vi "Modify Stage Limits.vi"(0 "Notifier Name":string, 5 "Limits":dbl[][](array[numeric]), 7 "Use Limits?":bool, 11 "Error In":errorcluster) -> (15 "Error Out":errorcluster)   [LabVIEW 2020]
uses:
  Stages Limits Type Defs/Stage Limits.ctl
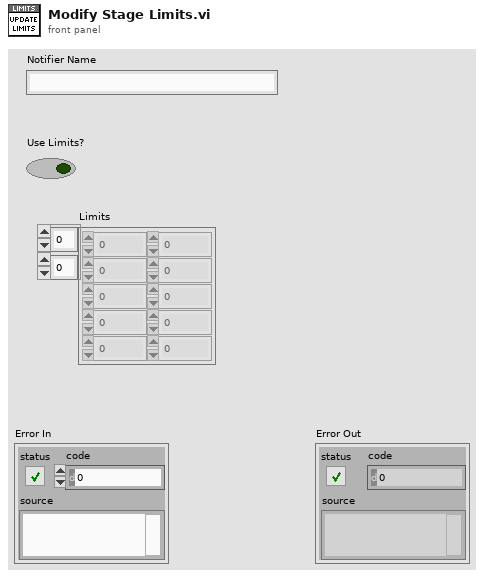
[diagram p1: front panel]
types:
  T1 = typedef "Stage Limits.ctl" = cluster{"Notifier":string, "Use Limits":bool, "Limits":dbl[][]}
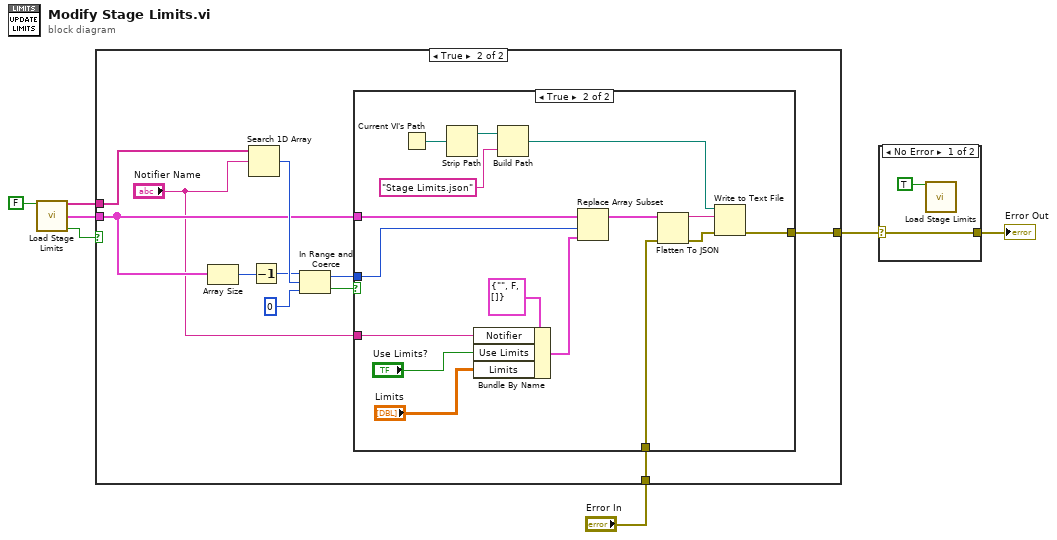
[diagram p0: block diagram]
diagram:
  n1 = call "Load Stage Limits.vi"("Update Limits"=FALSE) -> ("Notifier Names"=w6:string[], "Stage Limits"=w5:T1[], "Loaded"=w4:bool)  [unwired: 12 in]
  n2 = case shown="True" w4 {
    tunnel: w6 -> [_ w19]
    tunnel: w5 -> [_ w12]
    tunnel: [w8 w10] -> w3
    tunnel: "Error In" -> [w8 w9]
    frame False {
    }
    frame True {
      n3 = Array Size(array=w12) -> (size(s)=w16:i32)
      n4 = Search 1D Array(1D array=w19, element="Notifier Name") -> (index of element=w17:i32)  [unwired: 1 in]
      n5 = Decrement(x=w16) -> (x-1=w15:i32)
      n6 = In Range and Coerce(upper limit=w15, x=w17, lower limit=0) -> (coerced(x)=w13:i32, In Range?=w14:bool)
      n7 = case shown="True" w14 {
        tunnel: w13 -> [_ w35]
        tunnel: w12 -> [_ w36]
        tunnel: "Notifier Name" -> [_ w32]
        tunnel: [w20 w22] -> w10
        tunnel: w9 -> [w20 w21]
        frame False {
        }
        frame True {
          n8 = Current VI's Path() -> (path=w26:path)
          n9 = Strip Path(path=w26) -> (stripped path=w25:path)  [unwired: 1 out]
          n10 = Bundle By Name(cluster=T1 {"Notifier"="", "Use Limits"=FALSE, "Limits"=[]} ("Stage Limits"), "Notifier"=w32, "Use Limits"="Use Limits?", "Limits"="Limits") -> (w33:T1)
          n11 = Build Path(base path=w25, name or relative path="Stage Limits.json") -> (appended path=w23:path)
          n12 = Replace Array Subset(array=w36, new element=w33, index=w35) -> (w28:T1[])
          n13 = Flatten To JSON(anything=w28, error in (no error)=w21) -> (JSON string=w29:string, 11:w27:errorcluster)  [unwired: 1 in]
          n14 = Write to Text File(file (use dialog)=w23, text=w29, error in=w27) -> (error out=w22:errorcluster)  [unwired: 1 in, 2 out]
        }
      }
    }
  }
  n15 = case shown="No Error" w3 {
    selector: w3 -> [w37 w39]
    tunnel: [w37 w39] -> w2
    frame No Error {
      n16 = call "Load Stage Limits.vi"("Update Limits"=TRUE) -> ()  [unwired: 12 in, 3 out]
    }
    frame Error {
    }
  }
  "Error Out" <- w2
